vi "valueToInt.vi"(1 "variant":variant) -> (0 "data":i32)   [LabVIEW 2015]
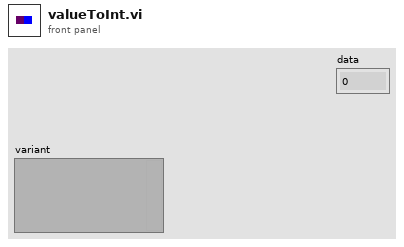
[diagram p1: front panel]
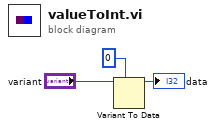
[diagram p0: block diagram]
diagram:
  n1 = Variant To Data(type=0, Variant="variant") -> (data=→"data":i32)  [unwired: 1 in, 1 out]
